vi "mV.vi"() -> ()   [LabVIEW 2026]
panel:
  out "Gain":string
  out "Frequency Amplifier IN":string
  out "Frequency Microphone OUT":string
  out "Vrms Amplifier IN":string
  out "Vrms Microphone OUT":string
  out "Vpp Headphone IN":string
  out "Vpp Amplifier OUT/Headphone IN -":string
  out "Vpp Amplifier OUT/Headphone IN +":string
  out "Vpp Amplifier IN":string
  out "Vpp Microphone OUT":string
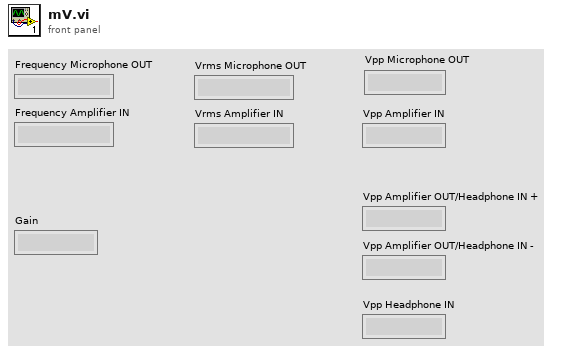
[diagram p1: front panel]
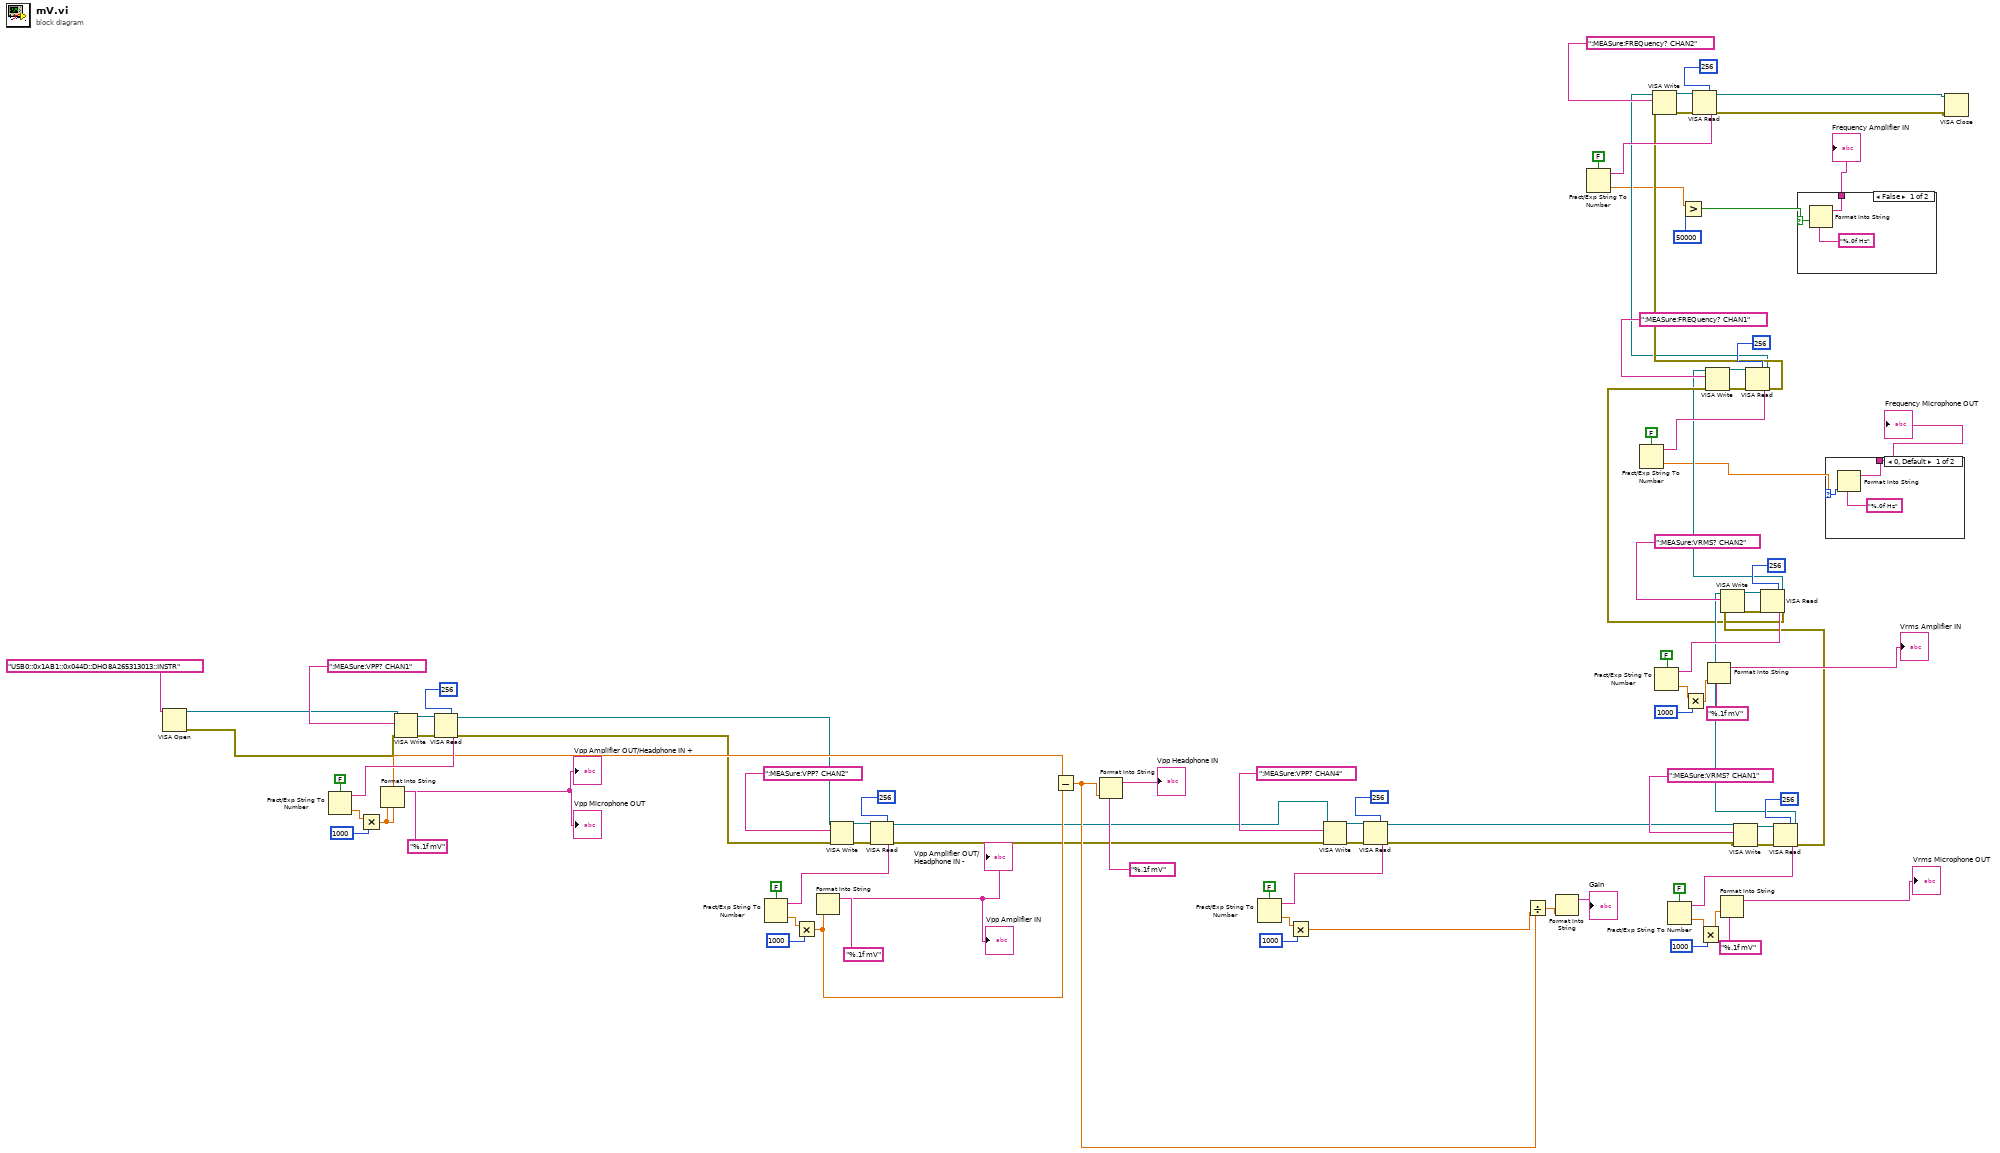
[diagram p0: block diagram]
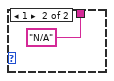
[diagram p2: hidden frame]
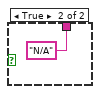
[diagram p3: hidden frame]
diagram:
  n1 = VISA Open(VISA resource name="USB0::0x1AB1::0x044D::DHO8A265313013::INSTR") -> (VISA resource name=w26:refnum<visa-resource-name>, error out=w27:errorcluster)  [unwired: 4 in]
  n2 = VISA Write(VISA resource name=w26, write buffer=":MEASure:VPP? CHAN1", error in (no error)=w27) -> (VISA resource name out=w93:refnum<visa-resource-name>, error out=w92:errorcluster)  [unwired: 1 out]
  n3 = VISA Read(VISA resource name=w93, byte count=256, error in (no error)=w92) -> (VISA resource name out=w19:refnum<visa-resource-name>, read buffer=w86:string, error out=w20:errorcluster)  [unwired: 1 out]
  n4 = Fract/Exp String To Number(use system decimal point (T)=FALSE, string=w86) -> (number=w85:dbl)  [unwired: 2 in, 1 out]
  n5 = Multiply(x=w85, y=1000) -> (x*y=w72:dbl)
  n6 = Format Into String(format string="%.1f mV", w72) -> (resulting string=→"Vpp Microphone OUT" →"Vpp Amplifier OUT/Headphone IN +":string)  [unwired: 2 in, 1 out]
  n7 = VISA Write(VISA resource name=w19, write buffer=":MEASure:VPP? CHAN2", error in (no error)=w20) -> (VISA resource name out=w83:refnum<visa-resource-name>, error out=w82:errorcluster)  [unwired: 1 out]
  n8 = VISA Read(VISA resource name=w83, byte count=256, error in (no error)=w82) -> (VISA resource name out=w18:refnum<visa-resource-name>, read buffer=w77:string, error out=w17:errorcluster)  [unwired: 1 out]
  n9 = Fract/Exp String To Number(use system decimal point (T)=FALSE, string=w77) -> (number=w76:dbl)  [unwired: 2 in, 1 out]
  n10 = Multiply(x=w76, y=1000) -> (x*y=w71:dbl)
  n11 = Format Into String(format string="%.1f mV", w71) -> (resulting string=→"Vpp Amplifier IN" →"Vpp Amplifier OUT/Headphone IN -":string)  [unwired: 2 in, 1 out]
  n12 = Subtract(x=w72, y=w71) -> (x-y=w24:dbl)
  n13 = Format Into String(format string="%.1f mV", w24) -> (resulting string=→"Vpp Headphone IN":string)  [unwired: 2 in, 1 out]
  n14 = VISA Write(VISA resource name=w18, write buffer=":MEASure:VPP? CHAN4", error in (no error)=w17) -> (VISA resource name out=w35:refnum<visa-resource-name>, error out=w34:errorcluster)  [unwired: 1 out]
  n15 = VISA Read(VISA resource name=w35, byte count=256, error in (no error)=w34) -> (VISA resource name out=w15:refnum<visa-resource-name>, read buffer=w30:string, error out=w16:errorcluster)  [unwired: 1 out]
  n16 = Fract/Exp String To Number(use system decimal point (T)=FALSE, string=w30) -> (number=w29:dbl)  [unwired: 2 in, 1 out]
  n17 = Multiply(x=w29, y=1000) -> (x*y=w25:dbl)
  n18 = Divide(x=w24, y=w25) -> (x/y=w23:dbl)
  n19 = Format Into String(w23) -> (resulting string=→"Gain":string)  [unwired: 3 in, 1 out]
  n20 = VISA Write(VISA resource name=w15, write buffer=":MEASure:VRMS? CHAN1", error in (no error)=w16) -> (VISA resource name out=w69:refnum<visa-resource-name>, error out=w68:errorcluster)  [unwired: 1 out]
  n21 = VISA Read(VISA resource name=w69, byte count=256, error in (no error)=w68) -> (VISA resource name out=w13:refnum<visa-resource-name>, read buffer=w64:string, error out=w14:errorcluster)  [unwired: 1 out]
  n22 = Fract/Exp String To Number(use system decimal point (T)=FALSE, string=w64) -> (number=w40:dbl)  [unwired: 2 in, 1 out]
  n23 = Multiply(x=w40, y=1000) -> (x*y=w39:dbl)
  n24 = Format Into String(format string="%.1f mV", w39) -> (resulting string=→"Vrms Microphone OUT":string)  [unwired: 2 in, 1 out]
  n25 = VISA Write(VISA resource name=w13, write buffer=":MEASure:VRMS? CHAN2", error in (no error)=w14) -> (VISA resource name out=w61:refnum<visa-resource-name>, error out=w60:errorcluster)  [unwired: 1 out]
  n26 = VISA Read(VISA resource name=w61, byte count=256, error in (no error)=w60) -> (VISA resource name out=w11:refnum<visa-resource-name>, read buffer=w56:string, error out=w12:errorcluster)  [unwired: 1 out]
  n27 = Fract/Exp String To Number(use system decimal point (T)=FALSE, string=w56) -> (number=w37:dbl)  [unwired: 2 in, 1 out]
  n28 = Multiply(x=w37, y=1000) -> (x*y=w36:dbl)
  n29 = VISA Write(VISA resource name=w11, write buffer=":MEASure:FREQuency? CHAN1", error in (no error)=w12) -> (VISA resource name out=w53:refnum<visa-resource-name>, error out=w52:errorcluster)  [unwired: 1 out]
  n30 = Format Into String(format string="%.1f mV", w36) -> (resulting string=→"Vrms Amplifier IN":string)  [unwired: 2 in, 1 out]
  n31 = VISA Read(VISA resource name=w53, byte count=256, error in (no error)=w52) -> (VISA resource name out=w9:refnum<visa-resource-name>, read buffer=w48:string, error out=w10:errorcluster)  [unwired: 1 out]
  n32 = Fract/Exp String To Number(use system decimal point (T)=FALSE, string=w48) -> (number=w2:dbl)  [unwired: 2 in, 1 out]
  n33 = VISA Write(VISA resource name=w9, write buffer=":MEASure:FREQuency? CHAN2", error in (no error)=w10) -> (VISA resource name out=w47:refnum<visa-resource-name>, error out=w46:errorcluster)  [unwired: 1 out]
  n34 = VISA Read(VISA resource name=w47, byte count=256, error in (no error)=w46) -> (VISA resource name out=w7:refnum<visa-resource-name>, read buffer=w42:string, error out=w8:errorcluster)  [unwired: 1 out]
  n35 = Fract/Exp String To Number(use system decimal point (T)=FALSE, string=w42) -> (number=w6:dbl)  [unwired: 2 in, 1 out]
  n36 = Greater?(x=w6, y=50000) -> (0:w4:bool)
  n37 = case shown="False" w4 {
    selector: w4 -> [w94 _]
    tunnel: [w96 "N/A"] -> w3
    frame False {
      n38 = Format Into String(format string="%.0f Hz", w94) -> (resulting string=w96:string)  [unwired: 2 in, 1 out]
    }
    frame True {
    }
  }
  "Frequency Amplifier IN" <- w3
  n39 = case shown="0, Default" w2 {
    selector: w2 -> [w98 _]
    tunnel: [w100 "N/A"] -> w1
    frame 0, Default {
      n40 = Format Into String(format string="%.0f Hz", w98) -> (resulting string=w100:string)  [unwired: 2 in, 1 out]
    }
    frame 1 {
    }
  }
  "Frequency Microphone OUT" <- w1
  n41 = VISA Close(VISA resource name=w7, error in (no error)=w8) -> ()  [unwired: 1 out]
